vi "Agilent 532XX Series Acquire Histogram.vi"() -> ()   [LabVIEW 2021]
doc: "This example shows how to acquire histogram using the VIs of the driver."
uses:
  <instrlib>/Agilent 532XX Series/Public/Configure/Measurement/Configure Measurement (Frequency).vi
  <instrlib>/Agilent 532XX Series/Agilent 532XX Series.lvlib
panel:
  in  "Auto Selection Number (100)":i32=100
  out "Number of Measurement":dbl
  out "Upper Range Value":dbl format="%#_12g"
  out "Lower Range Value":dbl format="%#_12g"
  out "Data":dbl[](array[numeric])
  in  "Point Number (100)":i32=100
  in  "Number of Measurement (100)":u32=100
  in  "Timeout (10000 ms)":u32=10000
  in  "VISA resource name":refnum<visa-resource-name>
  # "(c) 2010-2015 National Instruments.  ALL RIGHTS RESERVED."
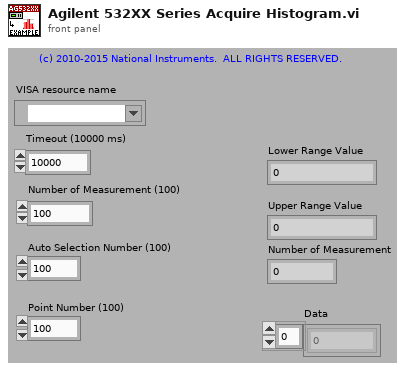
[diagram p1: front panel]
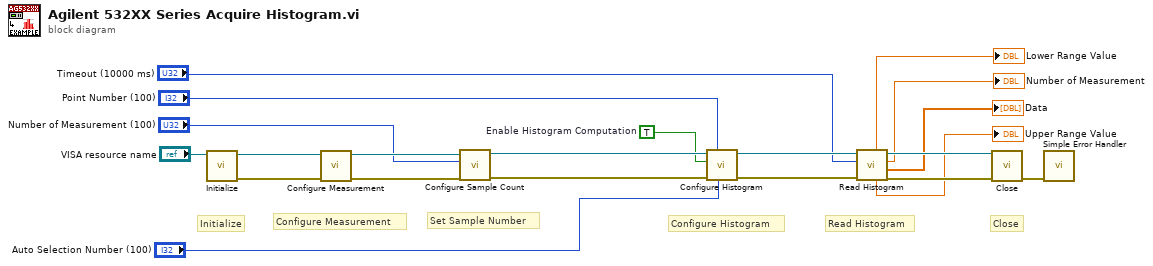
[diagram p0: block diagram]
diagram:
  w4 = TRUE  # Enable Histogram Computation
  # "Configure Histogram"
  # "Set Sample Number"
  # "Close"
  # "Read Histogram"
  # "Initialize"
  # "Configure Measurement"
  n1 = call <instrlib>:"Initialize.vi"("VISA resource name"="VISA resource name") -> ("error out"=w16:errorcluster, "VISA resource name out"=w15:refnum<visa-resource-name>)  [unwired: 3 in, 6 out]
  n2 = call-poly <instrlib>:"Configure Measurement.vi"("error in (no error)"=w16, "VISA resource name"=w15) -> ("error out"=w18:errorcluster, "VISA resource name out"=w19:refnum<visa-resource-name>)  [unwired: 3 in, 5 out]
  n3 = call <instrlib>:"Configure Sample Count.vi"("error in (no error)"=w18, "Sample Count (1)"="Number of Measurement (100)", "VISA resource name"=w19) -> ("error out"=w13:errorcluster, "VISA resource name out"=w14:refnum<visa-resource-name>)  [unwired: 7 out]
  n4 = call <instrlib>:"Configure Histogram.vi"("Auto Selection Number (100)"="Auto Selection Number (100)", "Point Number (100)"="Point Number (100)", "error in (no error)"=w13, "Enable Histogram Computation (T: Enable)"=w4, "VISA resource name"=w14) -> ("error out"=w1:errorcluster, "VISA resource name out"=w10:refnum<visa-resource-name>)  [unwired: 5 in]
  n5 = call <instrlib>:"Read Histogram.vi"("error in (no error)"=w1, "Timeout (10000 ms)"="Timeout (10000 ms)", "VISA resource name"=w10) -> ("error out"=w11:errorcluster, "Data"=→"Data":dbl[], "Number of Measurement"=→"Number of Measurement":dbl, "VISA resource name out"=w12:refnum<visa-resource-name>, "Upper Range Value"=→"Upper Range Value":dbl, "Lower Range Value"=→"Lower Range Value":dbl)  [unwired: 3 out]
  n6 = call <instrlib>:"Close.vi"("error in (no error)"=w11, "VISA resource name"=w12) -> ("error out"=w20:errorcluster)  [unwired: 9 out]
  n7 = call <vilib>:"Simple Error Handler.vi"("error in (no error)"=w20) -> ()  [unwired: 1 in, 8 out]
